vi "Register Modules in Event Manager--helper.vi"(7 "Application in":refnum<vi>, 8 "error in (no error)":errorcluster, 10 "New Modules":path[](array[path]), 11 "Modules IN":path[](array[path])) -> (0 "error out":errorcluster, 3 "Modules OUT":path[](array[path]))   [LabVIEW 2020, in "Event Manager.lvlib"]
doc: "____\nHAMPEL SOFTWARE ENGINEERING v2.6.0 (2023-12-19 10:54)"
uses:
  Event Manager.lvlib
  Libraries/hse-libraries/Source/hse-application/hse-application.lvclass/hse-application.ctl
  Libraries/hse-libraries/Source/hse-application/HSE Application not initialized--error.vi
  <vilib>/Utility/error.llb/Clear Errors.vi
  Libraries/hse-libraries/Source/hse-application/hse-application__GetSingleton.vi
  <vilib>/Utility/sysdir.llb/Get System Directory.vi
  <vilib>/Utility/error.llb/Error Cluster From Error Code.vi
  Libraries/hse-libraries/Source/hse-application/hse-application.lvclass
  Libraries/hse-libraries/Source/hse-dqmh/hse-dqmh-dynamicrequesters.lvlib
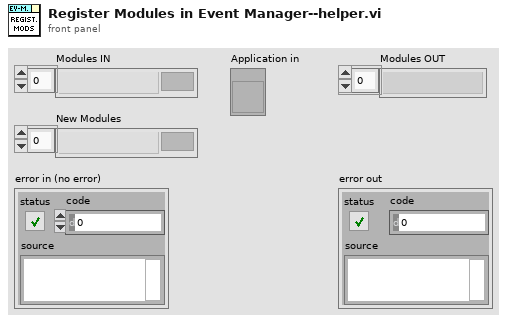
[diagram p1: front panel]
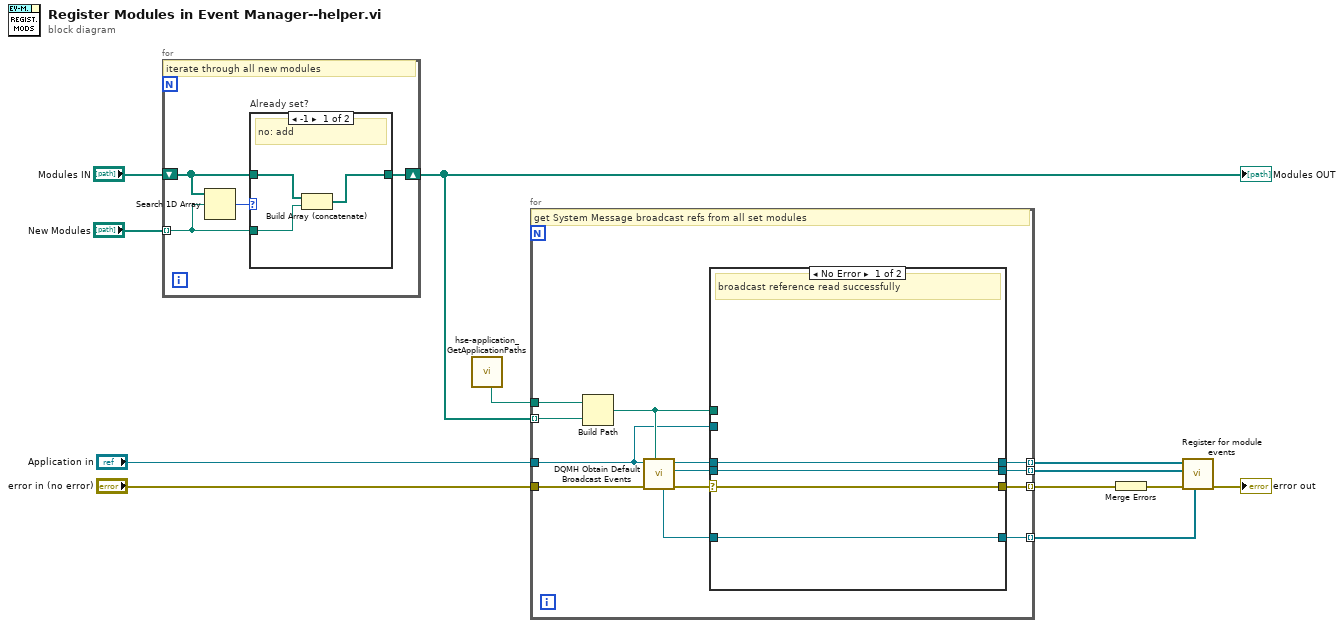
[diagram p0: block diagram]
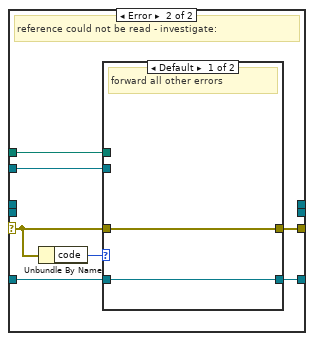
[diagram p3: hidden frame]
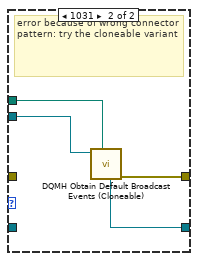
[diagram p4: hidden frame]
diagram:
  n1 = for {
    tunnel: "New Modules" -> [w13] mode=indexing
    shift-right: [w15] -> w3
    shift-left: "Modules IN" -> [w14]
    # "iterate through all new modules"
    n2 = Search 1D Array(1D array=w14, element=w13) -> (index of element=w16:i32)  [unwired: 1 in]
    n3 = case "Already set?" shown="-1" w16 {
      tunnel: [w17 w20] -> w15
      tunnel: w14 -> [w18 w20]
      tunnel: w13 -> [w19 _]
      frame -1 {
        # "no: add"
        n4 = Build Array (concatenate)(w18, w19) -> (w17:path[])
      }
      frame Default {
        # "yes: do nothing"
      }
    }
  }
  "Modules OUT" <- w3
  n5 = call "hse-application_GetApplicationPaths.vi"() -> ("Application Base Path"=w7:path)  [unwired: 5 in, 6 out]
  n6 = for {
    tunnel: w3 -> [w33] mode=indexing
    tunnel: w7 -> [w32]
    tunnel: "error in (no error)" -> [w31]
    tunnel: [w28] -> w9 mode=indexing
    tunnel: "Application in" -> [w25]
    tunnel: [w27] -> w6 mode=indexing
    tunnel: [w24] -> w5 mode=indexing
    tunnel: [w22] -> w4 mode=indexing
    # "get System Message broadcast refs from all set modules"
    n7 = Build Path(base path=w32, name or relative path=w33) -> (appended path=w26:path)
    n8 = call "DQMH Obtain Default Broadcast Events.vi"("Module Disk Path"=w26, "error in (no error)"=w31, "Application reference"=w25) -> ("error out"=w30:errorcluster, "Error Reported"=w21:refnum<user-event>, "Status Updated"=w23:refnum<user-event>, "System Message"=w29:refnum<user-event>)  [unwired: 3 in, 2 out]
    n9 = case shown="No Error" w30 {
      selector: w30 -> [w37 w39]
      tunnel: w29 -> [w36 w38]
      tunnel: [w37 w44] -> w28
      tunnel: [w36 w41] -> w27
      tunnel: w26 -> [_ w43]
      tunnel: w25 -> [_ w42]
      tunnel: [w35 _] -> w24
      tunnel: w23 -> [w35 _]
      tunnel: [w34 _] -> w22
      tunnel: w21 -> [w34 _]
      frame No Error {
        # "broadcast reference read successfully"
      }
      frame Error {
        # "reference could not be read - investigate:"
        n10 = Unbundle By Name(w39) -> ("code"=w40:i32)
        n11 = case shown="Default" w40 {
          tunnel: [w45 w50] -> w44
          tunnel: w43 -> [_ w49]
          tunnel: w42 -> [_ w48]
          tunnel: [w46 w47] -> w41
          tunnel: w39 -> [w45 _]
          tunnel: w38 -> [w46 _]
          frame Default {
            # "forward all other errors"
          }
          frame 1031 {
            # "error because of wrong connector pattern: try the cloneable variant"
            n12 = call "DQMH Obtain Default Broadcast Events (Cloneable).vi"("Module Disk Path"=w49, "Application reference"=w48) -> ("error out"=w50:errorcluster, "System Message"=w47:refnum<user-event>)  [unwired: 4 in, 4 out]
          }
        }
      }
    }
  }
  n13 = Merge Errors(w9) -> (w11:errorcluster)
  n14 = call "Register for module events.vi"("System Messages"=w6, "error in (no error)"=w11, "Errors"=w4, "Status Updates"=w5) -> ("error out"=→"error out":errorcluster)  [unwired: 7 in]
